vi "Socket.TCP Echo Client.vi"() -> ()   [LabVIEW 2014]
uses:
  Classes/Socket.TCP/Socket.TCP.lvclass
  <vilib>/Utility/error.llb/DialogType.ctl
panel:
  out "error out":errorcluster
  out "Stopping":bool
  out "Echoed from Server":string
  in  "String to send to Server (end with return)":string
  in  "Stop Button":bool
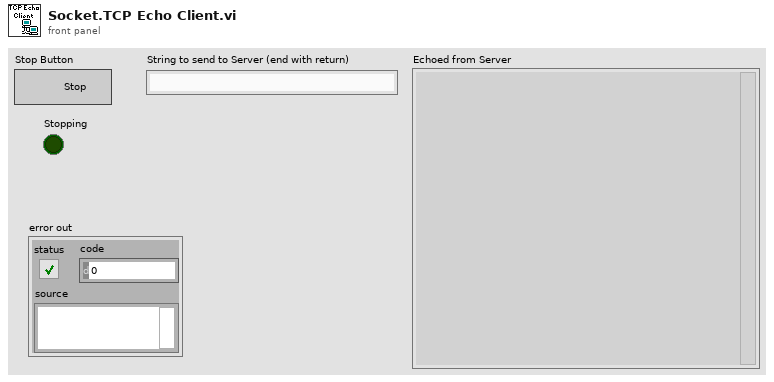
[diagram p1: front panel]
types:
  T1 = typedef "DialogType.ctl" = u16
  T2 = enum16{"Standard", "Buffered", "CRLF", "Immediate"}
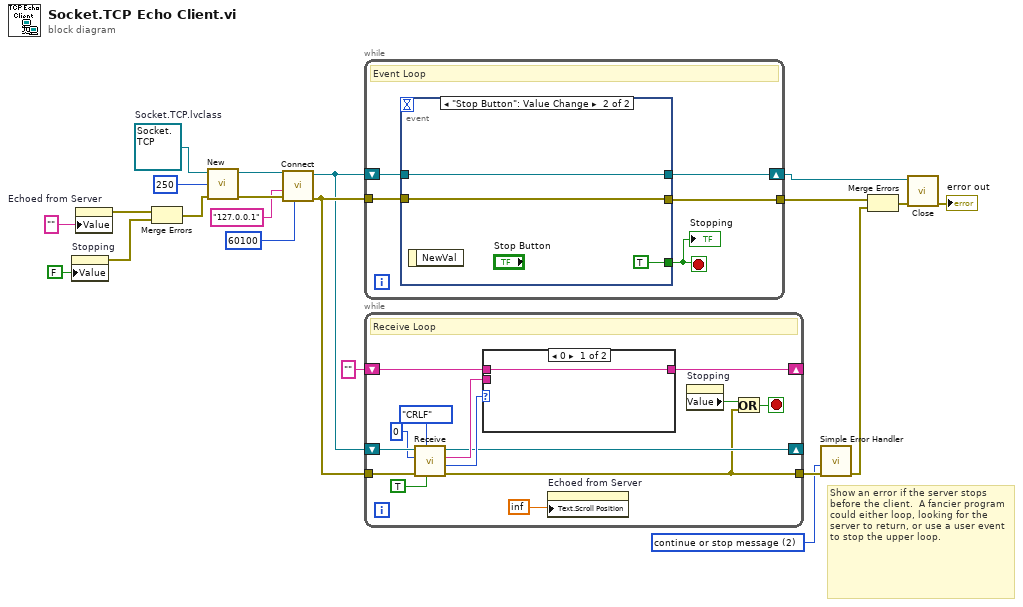
[diagram p0: block diagram]
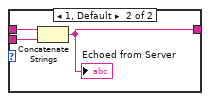
[diagram p2: hidden frame]
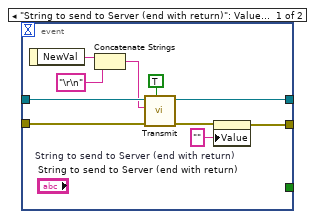
[diagram p3: hidden frame]
diagram:
  w5 = T1 2 items=["no dialog", "OK message", "continue or stop message", "OK message + warnings", "continue/stop + warnings"] ("type of dialog (OK msg:1)")
  w21 = refnum<class "Socket.TCP.lvclass"> refnum  # Socket.TCP.lvclass
  # "Show an error if the server stops before the client.  A fancier program could either loop, looking for the server to return, or use a user event to stop the upper loop."
  n1 = property on="Stopping" class="Bool (strict)"("Value"=FALSE ("Stopping")) -> (error out=w17:errorcluster)  [unwired: 2 in, 1 out]
  n2 = property on="Echoed from Server" class="Str"("Value"="" ("Echoed from Server")) -> (error out=w19:errorcluster)  [unwired: 2 in, 1 out]
  n3 = Merge Errors(w19, w17) -> (w15:errorcluster)
  n4 = call-dynamic "New.vi"("error in (no error)"=w15, "timeout"=250, "Socket.TCP in"=w21) -> ("error out"=w13:errorcluster, "Socket.TCP out"=w14:refnum<class "Socket.TCP.lvclass">)  [unwired: 7 in]
  n5 = call-dynamic "Connect.vi"("remote_port"=u16 60100, "error in (no error)"=w13, "remote_address"="127.0.0.1", "Socket.TCP in"=w14) -> ("error out"=w10:errorcluster, "Socket.TCP out"=w9:refnum<class "Socket.TCP.lvclass">)  [unwired: 6 in]
  n6 = while {
    tunnel: w10 -> [w25]
    tunnel: [w23] -> w1
    shift-right: [w22] -> w2
    shift-left: w9 -> [w26]
    stop <- w24 stop-if-true
    # "Event Loop"
    n7 = event shown="[1] \"Stop Button\": Value Change" {
      selector: _ -> [_ _]
      dyn-events: _ -> [_ _]
      timeout: _ -> [_ _]
      tunnel: w26 -> [w34 w38]
      tunnel: w25 -> [w33 w37]
      tunnel: [w28 w38] -> w22
      tunnel: [w27 w37] -> w23
      tunnel: [_ TRUE] -> w24
      event "String to send to Server (end with return)": Value Change {
        n8 = event-data() -> ("NewVal"=w35:string)  [unwired: 1 in]
        n9 = Concatenate Strings(w35, "\r\n" ("string")) -> (w32:string)
        n10 = call-dynamic "Transmit.vi"("packet? (f)"=TRUE, "error in (no error)"=w33, "data"=w32, "Socket.TCP in"=w34) -> ("error out"=w30:errorcluster, "Socket.TCP out"=w28:refnum<class "Socket.TCP.lvclass">)  [unwired: 5 in, 1 out]
        n11 = property on="String to send to Server (end with return)" class="Str"(error in=w30, "Value"="" ("String to send to Server (end with return)")) -> (error out=w27:errorcluster)  [unwired: 1 in, 1 out]
      }
      event "Stop Button": Value Change {
        n12 = event-data() -> ()  [unwired: 1 in, 1 out]
      }
    }
    "Stopping" <- w24
  }
  n13 = while {
    tunnel: w10 -> [w52]
    shift-right: [w47] -> _
    shift-left: w9 -> [w53]
    tunnel: [w42] -> w7
    shift-right: [w46] -> _
    shift-left: "" ("data out") -> [w45]
    stop <- w41 stop-if-true
    # "Receive Loop"
    n14 = call-dynamic "Receive.vi"("clear_timeout_error (f)"=TRUE, "mode (standard)"=T2."CRLF", "error in (no error)"=w52, "bufsize (0)"=u32 0, "Socket.TCP in"=w53) -> ("error out"=w42:errorcluster, "bytes_read"=w49:i32, "data_out"=w48:string, "Socket.TCP out"=w47:refnum<class "Socket.TCP.lvclass">)  [unwired: 3 in]
    n15 = case shown="0" w49 {
      tunnel: w48 -> [_ w57]
      tunnel: [w54 w56] -> w46
      tunnel: w45 -> [w54 w55]
      frame 0 {
      }
      frame 1, Default {
        n16 = Concatenate Strings(w55, w57) -> (w56:string)
        "Echoed from Server" <- w56
      }
    }
    n17 = property on="Echoed from Server" class="Str"("Text.Scroll Position"=inf) -> ()  [unwired: 2 in, 2 out]
    n18 = property on="Stopping" class="Bool (strict)"() -> ("Value"=w43:bool)  [unwired: 2 in, 2 out]
    n19 = Or(x=w43, y=w42) -> (x .or. y?=w41:bool)
  }
  n20 = call <vilib>:"Simple Error Handler.vi"("type of dialog (OK msg:1)"=w5, "error in (no error)"=w7) -> ("error out"=w6:errorcluster)  [unwired: 3 in, 4 out]
  n21 = Merge Errors(w1, w6) -> (w4:errorcluster)
  n22 = call-dynamic "Close.vi"("error in (no error)"=w4, "Socket.TCP in"=w2) -> ("error out"=→"error out":errorcluster)  [unwired: 8 in, 1 out]
